vi "Beta Function.vi"(10 "y":dbl format="%.2f", 11 "x":dbl format="%.2f") -> (3 "b(x, y)":dbl format="%.2f")   [LabVIEW 2010, in "NI_Gmath.lvlib"]
doc: "Evaluates the beta function or the incomplete beta function. You must manually select the polymorphic instance you want to use."
uses:
  NI_Gmath.lvlib
  lvanlys.dll
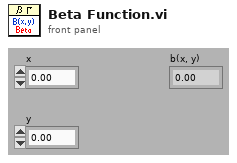
[diagram p1: front panel]
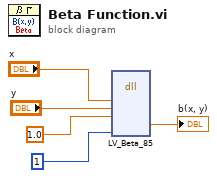
[diagram p0: block diagram]
diagram:
  n1 = dll-call lib="C:/Program Files/National Instruments/LabVIEW 2010/resource/lvanlys.*" fn="LV_Beta_85"("x"="x", "y"="y", "a"=1.0, "funcType"=1) -> ("beta(x,y,a)"=→"b(x, y)":dbl)  [unwired: 9 in, 2 out]
